vi "Write Nested Models.vi"(10 "Nested Models":refnum<class "IModel.lvclass">[](array[class]), 11 "IModel In":refnum<class "IModel.lvclass">) -> (3 "IModel Out":refnum<class "IModel.lvclass">)   [LabVIEW 2015, in "IModel.lvlib" / "IModel.lvclass"]
uses:
  IModel.lvclass
  IModel.lvclass/IModel.ctl
  IModel Messages/Launch Nested Models Msg/Launch Nested Models Msg.lvclass
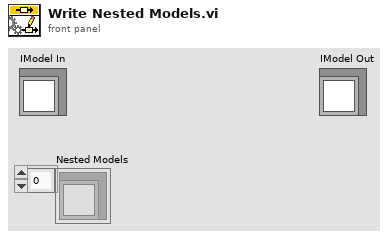
[diagram p1: front panel]
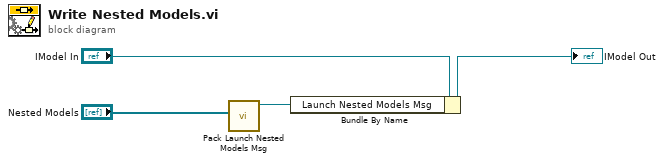
[diagram p0: block diagram]
diagram:
  n1 = call "Pack Launch Nested Models Msg.vi"("Models"="Nested Models") -> ("Launch Nested Models Msg"=w2:refnum<class "Launch Nested Models Msg.lvclass">)  [unwired: 10 in]
  n2 = Bundle By Name(cluster="IModel In", "Launch Nested Models Msg"=w2) -> (→"IModel Out":refnum<class "IModel.lvclass">)
